vi "Store Configuration Parameters.vi"(8 "error in (no error)":errorcluster, 10 "refnum":T1, 11 "Step Configuration in":refnum<class "Step Configuration.lvclass">) -> (0 "error out":errorcluster, 2 "refnum out":T1, 3 "Step Configuration out":refnum<class "Step Configuration.lvclass">)   [LabVIEW 2017, in "Measurement Actor.lvlib" / "Step Configuration.lvclass"]
uses:
  Step Configuration.lvclass
  C:/Program Files (x86)/National Instruments/LabVIEW 2017/user.lib/Configuration Dialog Actor/Configuration.lvclass
  <vilib>/Utility/config.llb/Config Data RefNum.ctl
  <userlib>/Configuration Dialog Actor/Configuration.lvclass/Configuration.ctl
  Step Configuration.lvclass/Step Configuration.ctl
  <userlib>/Configuration Dialog Actor/Configuration.lvclass
  Logger/config/Logger Configuration.lvclass
  <vilib>/Utility/config.llb/NI_LVConfig.lvlib
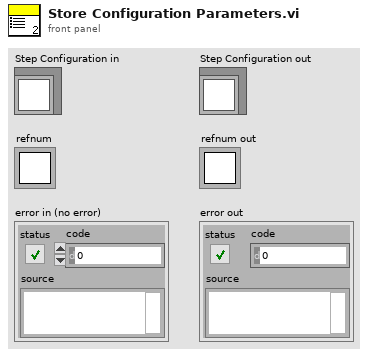
[diagram p1: front panel]
types:
  T1 = typedef "NI_LVConfig.lvlib/Config Data RefNum.ctl" = refnum<k1>
  T2 = cluster{"Run indefinitely":bool, "Iterations":i32}
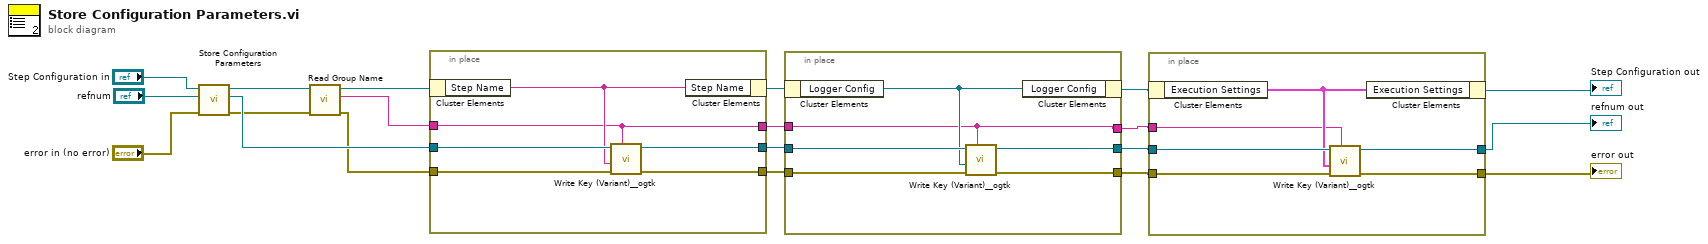
[diagram p0: block diagram]
diagram:
  n1 = call-parent "Store Configuration Parameters.vi"("error in (no error)"="error in (no error)", "refnum"="refnum", "Configuration in"="Step Configuration in") -> ("error out"=w12:errorcluster, "refnum out"=w17:T1, "Configuration out"=w13:refnum<class "Step Configuration.lvclass">)  [unwired: 6 in]
  n2 = call <userlib>:"Read Group Name.vi"("error in (no error)"=w12, "Configuration in"=w13) -> ("error out"=w10:errorcluster, "Group Name"=w9:string, "Configuration out"=w11:refnum<class "Step Configuration.lvclass">)  [unwired: 7 in]
  n3 = in-place {
    in-place-border: w17 -> [w26]
    in-place-border: [w25] -> w15
    in-place-border: [w24] -> w14
    in-place-border: w10 -> [w22]
    in-place-border: w9 -> [w21]
    in-place-border: [w21] -> w8
    n4 = in-place-cluster #1(w11) -> ("Step Name"=w23:string)
    n5 = call <userlib>:"Write Key (Variant)__ogtk.vi"("section"=w21, "error in (no error)"=w22, "key-value"=w23, "refnum"=w26) -> ("error out"=w24:errorcluster, "refnum out"=w25:T1)  [unwired: 6 in]
    n6 = in-place-cluster #1("Step Name"=w23) -> (w16:refnum<class "Step Configuration.lvclass">)
  }
  n7 = in-place {
    in-place-border: w15 -> [w32]
    in-place-border: [w31] -> w5
    in-place-border: [w30] -> w4
    in-place-border: w14 -> [w28]
    in-place-border: w8 -> [w27]
    in-place-border: [w27] -> w6
    n8 = in-place-cluster #2(w16) -> ("Logger Config"=w29:refnum<class "Logger Configuration.lvclass">)
    n9 = call <userlib>:"Write Key (Variant)__ogtk.vi"("section"=w27, "error in (no error)"=w28, "key-value"=w29, "refnum"=w32) -> ("error out"=w30:errorcluster, "refnum out"=w31:T1)  [unwired: 6 in]
    n10 = in-place-cluster #2("Logger Config"=w29) -> (w7:refnum<class "Step Configuration.lvclass">)
  }
  n11 = in-place {
    in-place-border: w5 -> [w38]
    in-place-border: [w37] -> w2
    in-place-border: [w36] -> w3
    in-place-border: w4 -> [w34]
    in-place-border: w6 -> [w33]
    n12 = in-place-cluster #3(w7) -> ("Execution Settings"=w35:T2)
    n13 = call <userlib>:"Write Key (Variant)__ogtk.vi"("section"=w33, "error in (no error)"=w34, "key-value"=w35, "refnum"=w38) -> ("error out"=w36:errorcluster, "refnum out"=w37:T1)  [unwired: 6 in]
    n14 = in-place-cluster #3("Execution Settings"=w35) -> (→"Step Configuration out":refnum<class "Step Configuration.lvclass">)
  }
  "error out" <- w3
  "refnum out" <- w2
